vi "PD250 PWM.vi"(8 "Board Selector":T1, 9 "HMP4040_IN":refnum<visa-resource-name>, 10 "Message IN":string=" ") -> (0 "error out":errorcluster, 1 "Result (bool)":bool, 2 "Message OUT":string, 3 "ControlBoard OUT":refnum<visa-resource-name>)   [LabVIEW 2022 SP3]
uses:
  Serial Board Com/Board Select.ctl
  HMP4000 Communication/HMP4040_ChannelControl.ctl
  <vilib>/DAQmx/read.llb/DAQmx Read (Analog 1D Wfm NChan NSamp).vi
  <vilib>/DAQmx/miscellaneous.llb/DAQmx Fill In Error Info.vi
panel:
  in  "error in (no error) 2":errorcluster
  out "Duty Cycle VISA Write":string[](array[string])
  out "Analysis Leg":i32
  in  "Debug Mode":bool
  out "Waveforms":T2
  out "Active Leg":i32
  out "Result (color)":u32(colorbox)
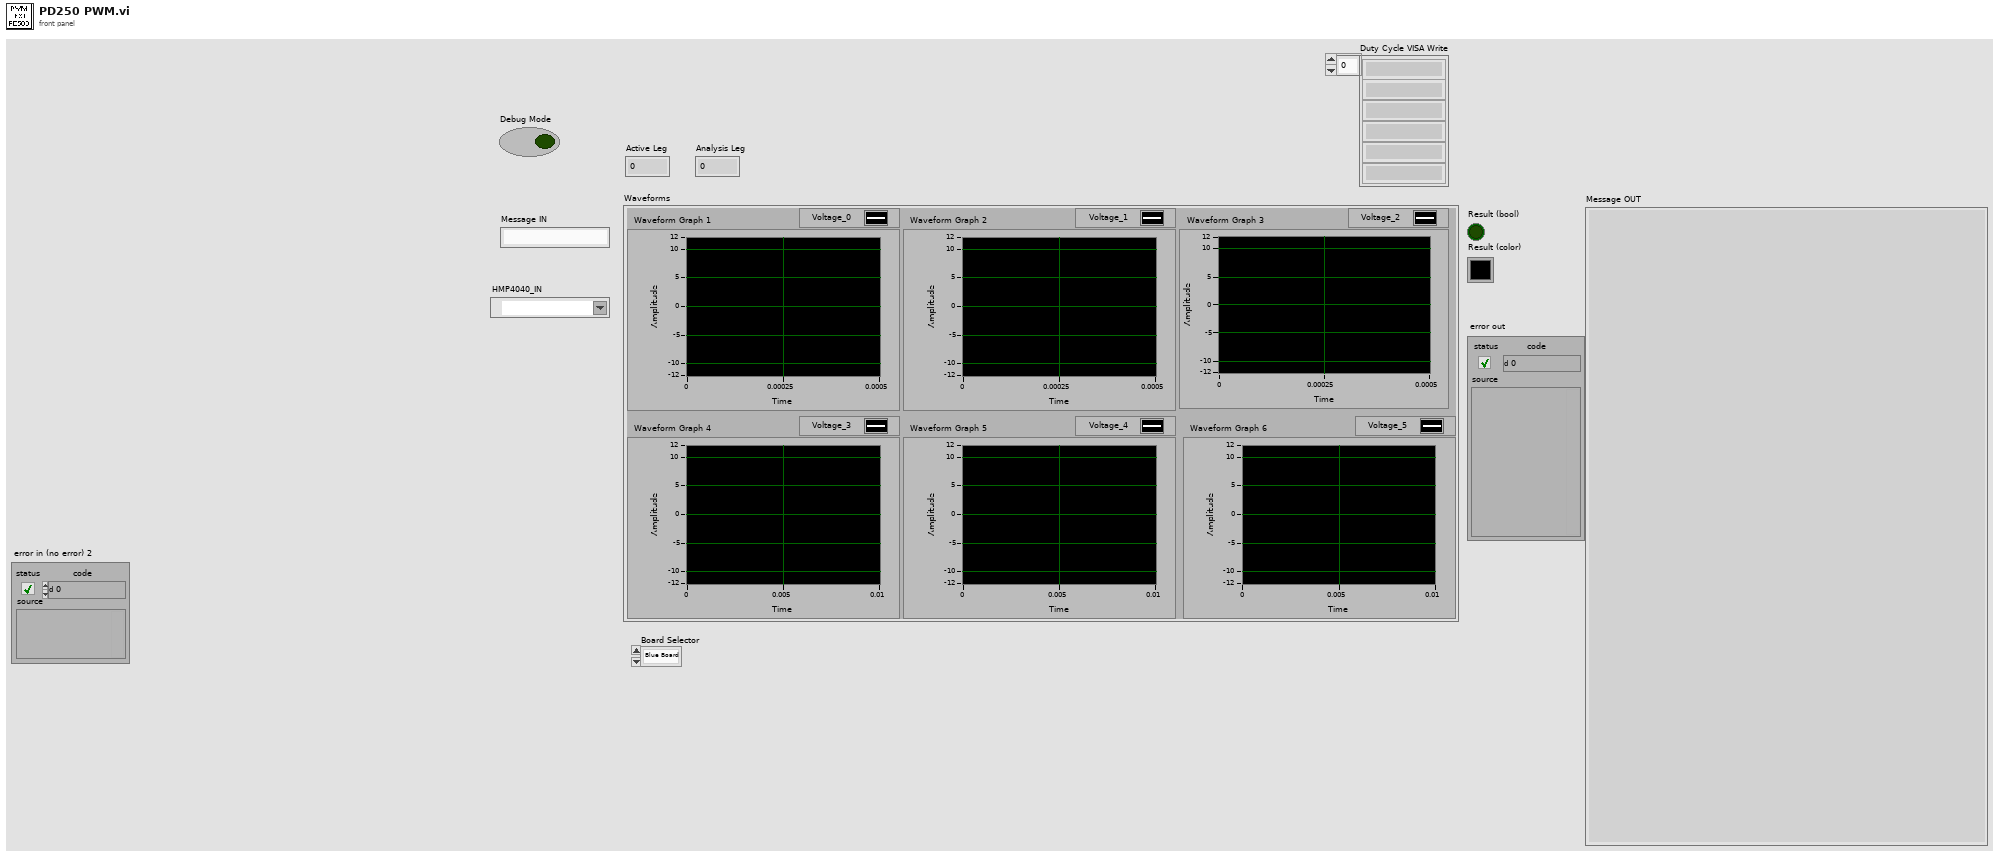
[diagram p1: front panel]
types:
  T1 = typedef "Board Select.ctl" = enum16{"Blue Board", "Green Board"}
  T2 = cluster{"Waveform Graph 1":waveform(dbl), "Waveform Graph 2":waveform(dbl), "Waveform Graph 3":waveform(dbl), "Waveform Graph 4":waveform(dbl), "Waveform Graph 5":waveform(dbl), "Waveform Graph 6":waveform(dbl)}
  T3 = typedef "HMP4040_ChannelControl.ctl" = cluster{"CH1 Voltage":dbl, "CH1 Current":dbl, "CH1 Output":bool, "CH2 Voltage":dbl, "CH2 Current":dbl, "CH2 Output":bool, "CH3 Voltage":dbl, "CH3 Current":dbl, "CH3 Output":bool, "CH4 Voltage":dbl, "CH4 Current":dbl, "CH4 Output":bool, "Master Output":bool}
  T4 = cluster{"data[0]":waveform(dbl), "data[1]":waveform(dbl), "data[2]":waveform(dbl), "data[3]":waveform(dbl), "data[4]":waveform(dbl), "data[5]":waveform(dbl)}
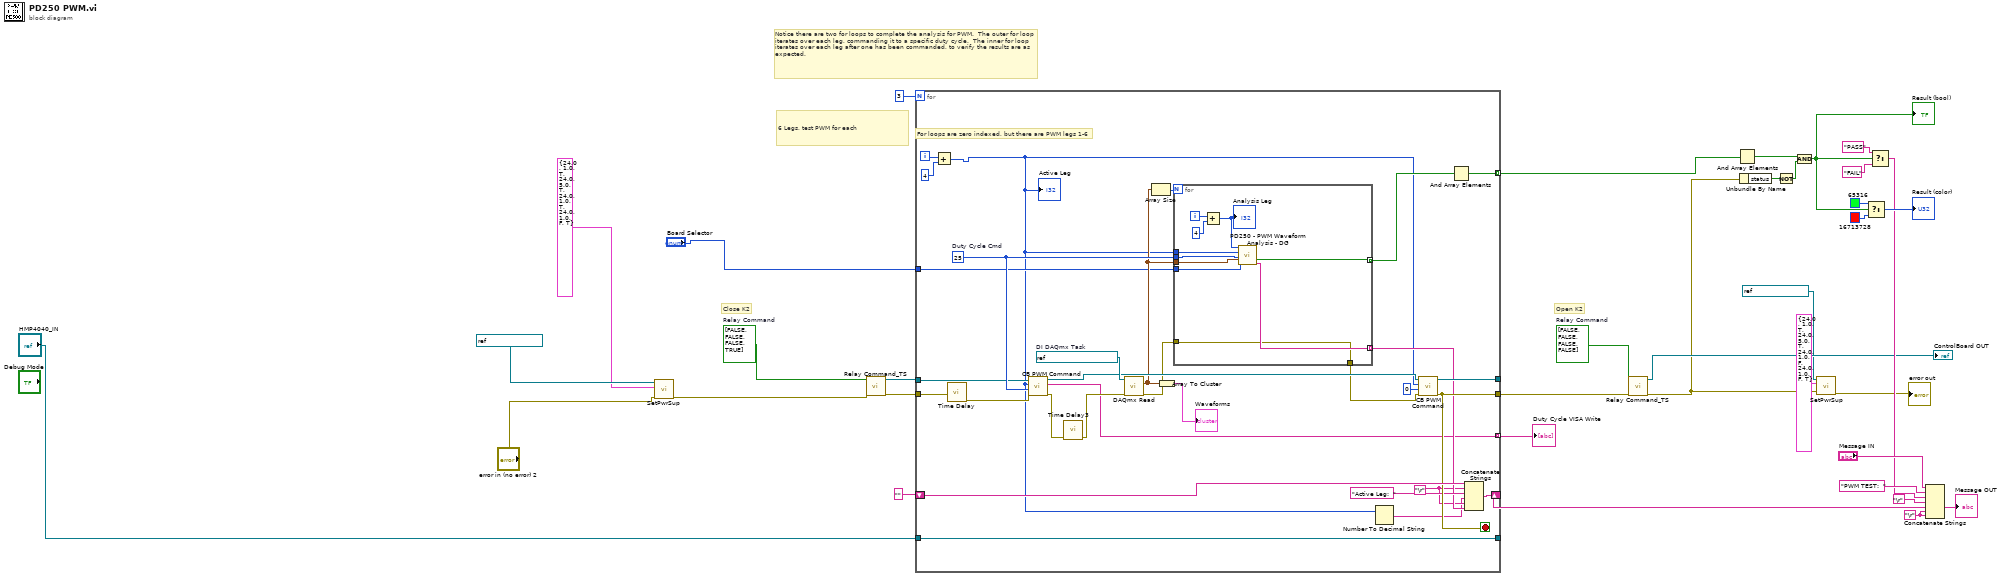
[diagram p0: block diagram]
diagram:
  w11 = bool[] [FALSE, FALSE, FALSE, TRUE]  # Relay Command
  w1 = bool[] [FALSE, FALSE, FALSE, FALSE]  # Relay Command
  w25 = "\r"
  # "Close K2"
  # "Open K2"
  # "Notice there are two for loops to complete the analysis for PWM.  The outer for loop iterates over each leg, commanding it to a specific duty cycle.  The inner for loop iterates over each leg after one has been commanded, to verify the results are as expected."
  # "6 Legs, test PWM for each"
  n1 = call "SetPwrSup.vi"("error in (no error)"="error in (no error) 2", "HMP4040 Channel Settings"=T3 {"CH1 Voltage"=24.0, "CH1 Current"=1.0, "CH1 Output"=TRUE, "CH2 Voltage"=24.0, "CH2 Current"=5.0, "CH2 Output"=TRUE, "CH3 Voltage"=24.0, "CH3 Current"=1.0, "CH3 Output"=TRUE, "CH4 Voltage"=24.0, "CH4 Current"=1.0, "CH4 Output"=FALSE, "Master Output"=TRUE}, "HMP4040 IN"=refnum<visa-resource-name> "HMP4040_FTS2" ("VISA resource name")) -> ("error out"=w7:errorcluster)  [unwired: 7 in, 1 out]
  n2 = call "Relay Command_TS.vi"("error in (no error)"=w7, "Relay Command"=w11) -> ("error out"=w13:errorcluster, "VISA Refnum out"=w15:refnum<visa-resource-name>)  [unwired: 8 in]
  n3 = for {
    N: 3 -> [_]
    tunnel: [w66] -> w36 mode=indexing
    shift-right: [w64] -> w23
    shift-left: "" -> [w63]
    tunnel: [w59] -> _
    tunnel: "HMP4040_IN" -> [w59]
    tunnel: [w58] -> w17
    tunnel: [w53] -> _
    tunnel: w13 -> [w43]
    tunnel: w15 -> [w48]
    tunnel: [w45] -> w12 mode=indexing
    tunnel: "Board Selector" -> [w44]
    i -> [w39]
    stop <- w58 stop-if-true
    w50 = "\r"
    w60 = 25  # Duty Cycle Cmd
    w65 = refnum<k21> "FTS2_PWMInput_DG"  # DI DAQmx Task
    # "For loops are zero indexed, but there are PWM legs 1-6"
    n4 = Add(x=w39, y=4) -> (x+y=w38:i32)
    "Active Leg" <- w38
    n5 = call "Time Delay"("error in (no error)"=w43) -> ("error out"=w42:errorcluster)  [unwired: 10 in]
    n6 = call "CB PWM Command.vi"("error in (no error)"=w42, "Duty Cycle"=w60, "Leg"=w38, "VISA Refnum in"=w48) -> ("error out"=w47:errorcluster, "read buffer"=w45:string, "VISA Refnum out"=w61:refnum<visa-resource-name>)  [unwired: 5 in]
    n7 = call "Time Delay3"("error in (no error)"=w47) -> ("error out"=w46:errorcluster)  [unwired: 10 in]
    n8 = call-poly <vilib>:"DAQmx Read.vi"("task/channels in"=w65, "error in"=w46) -> ("data"=w54:waveform(dbl)[], "error out"=w40:errorcluster)  [unwired: 11 in, 1 out]
    n9 = Array Size(array=w54) -> (size(s)=w55:i32)
    n10 = Array To Cluster(array=w54) -> (cluster=→"Waveforms":T4)
    n11 = for {
      N: w55 -> [_]
      tunnel: w60 -> [w76]
      tunnel: w54 -> [w75]
      tunnel: w38 -> [w74]
      tunnel: [w73] -> w56 mode=indexing
      tunnel: [w72] -> w51 mode=indexing
      tunnel: w44 -> [w71]
      tunnel: [w70] -> w41
      tunnel: w40 -> [w70]
      i -> [w69]
      n12 = Add(x=w69, y=4) -> (x+y=w67:i32)
      "Analysis Leg" <- w67
      n13 = call "PD250 - PWM Waveform Analysis - DG.vi"("Analysis Leg"=w67, "Active Leg"=w74, "Duty Cycle"=w76, "Waveform"=w75, "Board Selector"=w71) -> ("Result (Boolean)"=w73:bool, "Message"=w72:string)  [unwired: 9 in]
    }
    n14 = Number To Decimal String(number=w38) -> (decimal integer string=w49:string)  [unwired: 1 in]
    n15 = call "CB PWM Command.vi"("error in (no error)"=w41, "Duty Cycle"=0, "Leg"=w38, "VISA Refnum in"=w61) -> ("error out"=w58:errorcluster, "VISA Refnum out"=w53:refnum<visa-resource-name>)  [unwired: 5 in, 1 out]
    n16 = And Array Elements(Boolean array=w56) -> (logical AND=w66:bool)
    n17 = Concatenate Strings(w63, w50, "Active Leg:  ", w49, w50, w51) -> (w64:string)
  }
  "Duty Cycle VISA Write" <- w12
  n18 = call "Relay Command_TS.vi"("error in (no error)"=w17, "Relay Command"=w1) -> ("error out"=w4:errorcluster, "VISA Refnum out"=→"ControlBoard OUT":refnum<visa-resource-name>)  [unwired: 8 in]
  n19 = And Array Elements(Boolean array=w36) -> (logical AND=w26:bool)
  n20 = Unbundle By Name(w4) -> ("status"=w29:bool)
  n21 = Not(x=w29) -> (.not. x?=w28:bool)
  n22 = And(x=w26, y=w28) -> (x .and. y?=w27:bool)
  "Result (bool)" <- w27
  n23 = call "SetPwrSup.vi"("error in (no error)"=w4, "HMP4040 Channel Settings"=T3 {"CH1 Voltage"=24.0, "CH1 Current"=1.0, "CH1 Output"=TRUE, "CH2 Voltage"=24.0, "CH2 Current"=5.0, "CH2 Output"=TRUE, "CH3 Voltage"=24.0, "CH3 Current"=1.0, "CH3 Output"=FALSE, "CH4 Voltage"=24.0, "CH4 Current"=1.0, "CH4 Output"=FALSE, "Master Output"=TRUE}, "HMP4040 IN"=refnum<visa-resource-name> "HMP4040_FTS2" ("VISA resource name")) -> ("error out"=→"error out":errorcluster)  [unwired: 7 in, 1 out]
  n24 = Select(t=u32 65316 ("Result (color)"), s=w27, f=u32 16713728 ("Result (color)")) -> (s? t:f=→"Result (color)":u32)
  n25 = Select(t="PASS", s=w27, f="FAIL") -> (s? t:f=w18:string)
  n26 = Concatenate Strings("Message IN", "PWM TEST:  ", w18, "\r", w23, w25, w25) -> (→"Message OUT":string)
